vi "calibration.vi"(8 "graph error in":errorcluster, 10 "reference":refnum<vi>, 11 "Camera Session In":T1="cam0") -> (0 "graph error out":errorcluster, 3 "Camera Session out":T1)   [LabVIEW 2014]
uses:
  <vilib>/userdefined/High Color/IMAQdx.ctl
  <resource>/objmgr/imaqdx.rc
panel:
  out "Camera error in  2":errorcluster
  in  "x-axis calibration":T2={"1 px correlates to"=0.7298, "Min. Value"=280.0} {"Min. Value" min=0.0 max=2000.0 step=0.0001 format="%.4f"; "1 px correlates to" min=0.0 max=20.0 step=0.0001 format="%.4f"}
  in  "y-axis calibration":T3={"Vertical Pixel Size"=5.5, "focal length lens 1 (f1)"=60.0, "focal length lens 2 (f2)"=60.0} {"focal length lens 2 (f2)" min=0.0 max=1000.0 step=0.1 format="%.1f"; "focal length lens 1 (f1)" min=0.0 max=1000.0 step=0.1 format="%.1f"; "Vertical Pixel Size" min=0.0 max=20.0 step=0.1 format="%.1f"}
  in  "Cancel Button":bool
  in  "OK Button":bool
  in  "Camera error in":errorcluster
  out "Output":T4 {"Magnification of Optical System" format="%#_2g"}
  # "nm"
  # "According to your calculations, 1 px correlates to how many nanometers?"
  # "nm"
  # "µm"
  # "mm"
  # "mm"
  # "Properties:"
  # "px"
  # "px"
  # "x-axis:"
  # "nm"
  # "nm"
  # "y-axis:"
  # "mm"
  # "mm"
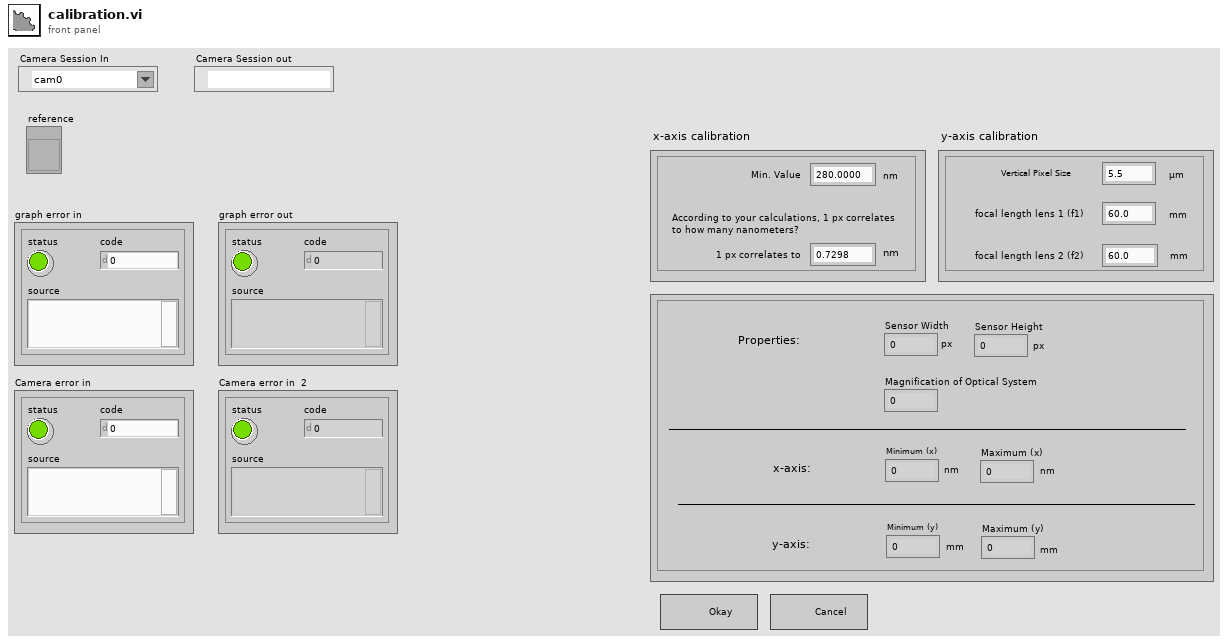
[diagram p1: front panel]
types:
  T1 = typedef "IMAQdx.ctl" = refnum<k21>
  T2 = cluster{"1 px correlates to":dbl, "Min. Value":dbl}
  T3 = cluster{"Vertical Pixel Size":dbl, "focal length lens 1 (f1)":dbl, "focal length lens 2 (f2)":dbl}
  T4 = cluster{"Magnification of Optical System":dbl, "Sensor Width":u32, "Sensor Height":u32, "Minimum (x)":dbl, "Maximum (x)":dbl, "Minimum (y)":dbl, "Maximum (y)":dbl}
  T5 = cluster{dbl, "Width":u32, "Height":u32, "Min. Value":dbl, dbl, "Y Scale.Range:Minimum":dbl, dbl}
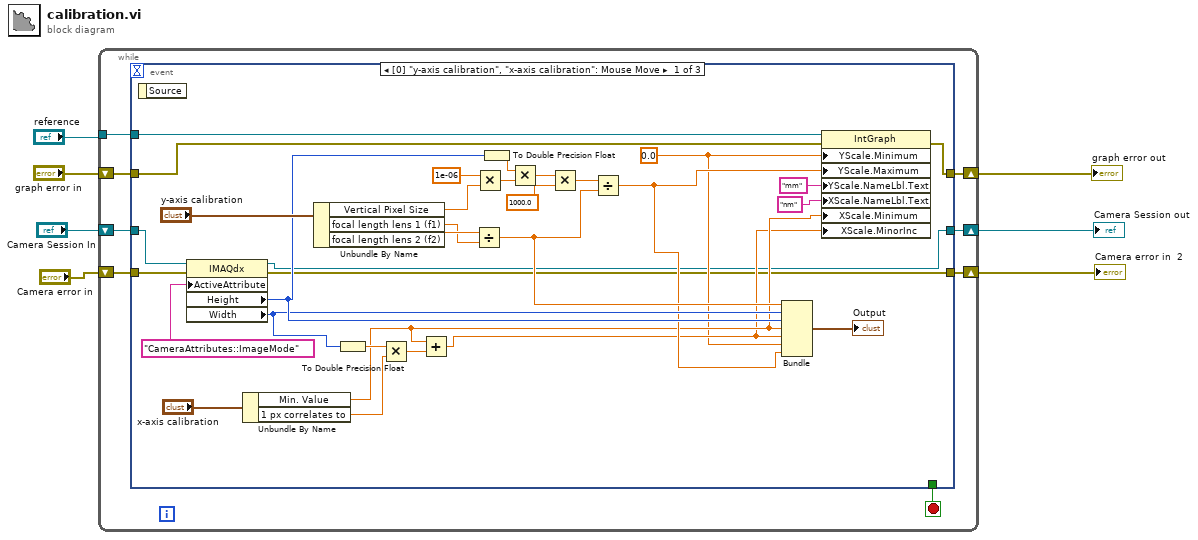
[diagram p0: block diagram]
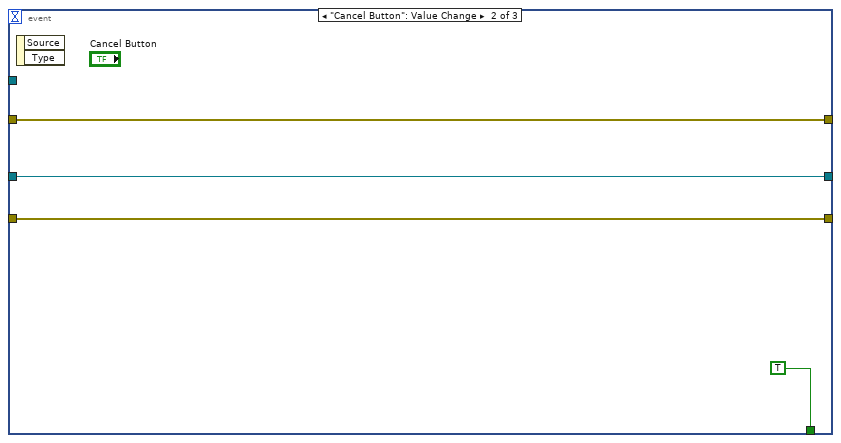
[diagram p2: hidden frame]
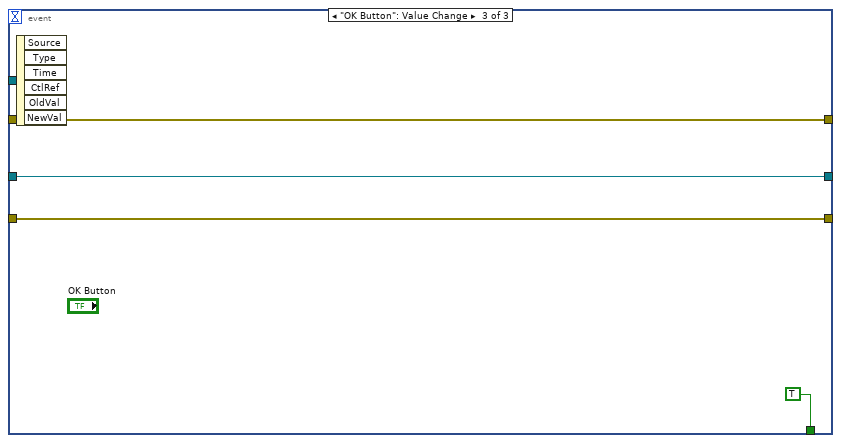
[diagram p3: hidden frame]
diagram:
  n1 = while {
    shift-right: [w14] -> w1
    shift-left: "graph error in" -> [w11]
    shift-right: [w13] -> w2
    shift-left: "Camera Session In" -> [w10]
    shift-right: [w12] -> w3
    shift-left: "Camera error in" -> [w9]
    tunnel: "reference" -> [w8]
    stop <- w15 stop-if-true
    n2 = event shown="[0] \"y-axis calibration\", \"x-axis calibration\": Mouse Move" {
      selector: _ -> [_ _ _]
      dyn-events: _ -> [_ _ _]
      timeout: _ -> [_ _ _]
      tunnel: w11 -> [w43 w51 w52]
      tunnel: [w42 w51 w52] -> w14
      tunnel: w10 -> [w41 w48 w53]
      tunnel: w9 -> [w40 w49 w54]
      tunnel: [_ TRUE TRUE] -> w15
      tunnel: [w18 w48 w53] -> w13
      tunnel: [w17 w49 w54] -> w12
      tunnel: w8 -> [w16 _ _]
      event "y-axis calibration", "x-axis calibration": Mouse Move {
        w19 = 0.0 ("Y Scale.Range:Minimum")
        n3 = event-data() -> ()  [unwired: 1 in, 1 out]
        n4 = property class="IMAQdx"(reference=w41, error in=w40, "ActiveAttribute"="CameraAttributes::ImageMode") -> (reference out=w18:T1, error out=w17:errorcluster, "Height"=w30:u32, "Width"=w25:u32)
        n5 = Unbundle By Name("x-axis calibration") -> ("Min. Value"=w21:dbl, "1 px correlates to"=w27:dbl)
        n6 = Unbundle By Name("y-axis calibration") -> ("Vertical Pixel Size"=w35:dbl, "focal length lens 1 (f1)"=w33:dbl, "focal length lens 2 (f2)"=w34:dbl)
        n7 = To Double Precision Float(number=w25) -> (double precision float=w26:dbl)
        n8 = Multiply(x=w26, y=w27) -> (x*y=w24:dbl)
        n9 = Add(x=w21, y=w24) -> (x+y=w20:dbl)
        n10 = Divide(x=w34, y=w33) -> (x/y=w31:dbl)
        n11 = Multiply(x=1e-06 ("y"), y=w35) -> (x*y=w45:dbl)
        n12 = To Double Precision Float(number=w30) -> (double precision float=w44:dbl)
        n13 = Multiply(x=w44, y=w45) -> (x*y=w39:dbl)
        n14 = Multiply(x=w39, y=1000.0) -> (x*y=w32:dbl)
        n15 = Divide(x=w32, y=w31) -> (x/y=w23:dbl)
        n16 = Bundle(w31, "Width"=w25, "Height"=w30, "Min. Value"=w21, w20, "Y Scale.Range:Minimum"=w19, w23) -> (→"Output":T5)  [unwired: 1 in]
        n17 = property on="Property Node" class="IntGraph"(reference=w16, error in=w43, "YScale.Minimum"=w19, "YScale.Maximum"=w23, "YScale.NameLbl.Text"="mm" ("Y Scale.Name Label.Text"), "XScale.NameLbl.Text"="nm" ("Y Scale.Name Label.Text"), "XScale.Minimum"=w21, "XScale.MinorInc"=w20) -> (error out=w42:errorcluster)  [unwired: 1 out]
      }
      event "Cancel Button": Value Change {
        n18 = event-data() -> ()  [unwired: 1 in, 2 out]
      }
      event "OK Button": Value Change {
        n19 = event-data() -> ()  [unwired: 1 in, 6 out]
      }
    }
  }
  "graph error out" <- w1
  "Camera Session out" <- w2
  "Camera error in  2" <- w3
